vi "Main (NoVisionRequired).vi"() -> ()   [LabVIEW 2019]
uses:
  3D utilities/3DS Models.ctl
  typedefs/System States.ctl
  typedefs/Render States.ctl
  <vilib>/picture/3D Picture Control/Old 3D Toolkit.llb/model.ctl
  <vilib>/picture/3D Picture Control/Old 3D Toolkit.llb/point3f.ctl
  <vilib>/picture/3D Picture Control/Old 3D Toolkit.llb/VertexMode.ctl
  XRay Cabinet/XRay Cabinet.lvclass
  C:/Users/Andrey/Documents/GitHub/XRaySimulatorLV/XRay Scene/XRay Scene.lvclass
  XRay Beam/XRay Beam.lvclass
  XRay CArm/XRay CArm.lvclass
  XRay Part Sample/XRay Part Sample.lvclass
  XRay Table/XRay Table.lvclass
  XRay Beam/XRay Beam.lvclass/XRay Beam.ctl
  XRay Part Sample/XRay Part Sample.lvclass/XRay Part Sample.ctl
  XRay Table/XRay Table.lvclass/XRay Table.ctl
  <vilib>/Analysis/coordinate.llb/3D Cartesian Coordinate Rotation (Euler) (Scalar).vi
  67ea9b9f-5008-4843-b879-74d7c71b0f0c.vi
  XRay Axis Rails/XRay Axis Rails.lvclass
  <vilib>/picture/3D Picture Control/Object/Create Object.vi
  <vilib>/picture/3D Picture Control/Object/Create Object (name).vi
  <vilib>/picture/3D Picture Control/Geometries/Create 3D Axis.vi
  <vilib>/picture/3D Picture Control/Object/Add Object.vi
  <vilib>/picture/3D Picture Control/Object/Add Object (no reference).vi
  XRay Scene/XRay Scene.lvclass
  <vilib>/Analysis/NI_AALPro.lvlib
  3D utilities/3D utilities.lvlib
  <vilib>/picture/3D Picture Control/NI_Old 3D Toolkit.lvlib
  LV_3D_Util64.dll
panel:
  out "XRay Image":sgl[][](graph)
  in  "Link to Z":bool
  in  "Mode":T1(ring)=enum."Wireframe"
  in  "High Res Render":bool
  in  "Play Button":bool
  in  "Reset":bool
  out "Render":bool
  in  "stop":bool
  in  "Part Angle":dbl(knob) caption="Part\nAngle"
  in  "Model":T2
  in  "FDD":sgl(slide)=11.031496 scale=1.0..15.0
  in  "DDA SIZE":sgl(slide)=2.003937 scale=1.0..4.0
  out "Size":i32=1240
  out "Time, ms":dbl=63.153
  out "Max Thickness":sgl=0.5478592
  in  "Y Position":dbl(slide)=7.0 scale=1.0..12.0
  in  "X Position":dbl(slide)=0.5 scale=-2.0..2.0
  in  "C Arm Angle":dbl(knob) caption="C-Arm\nAngle" scale=90.0..-90.0
  in  "Z position":sgl(slide)=4.0 scale=0.0..10.0
  out "3D Picture":refnum<vi>(3d-picture)
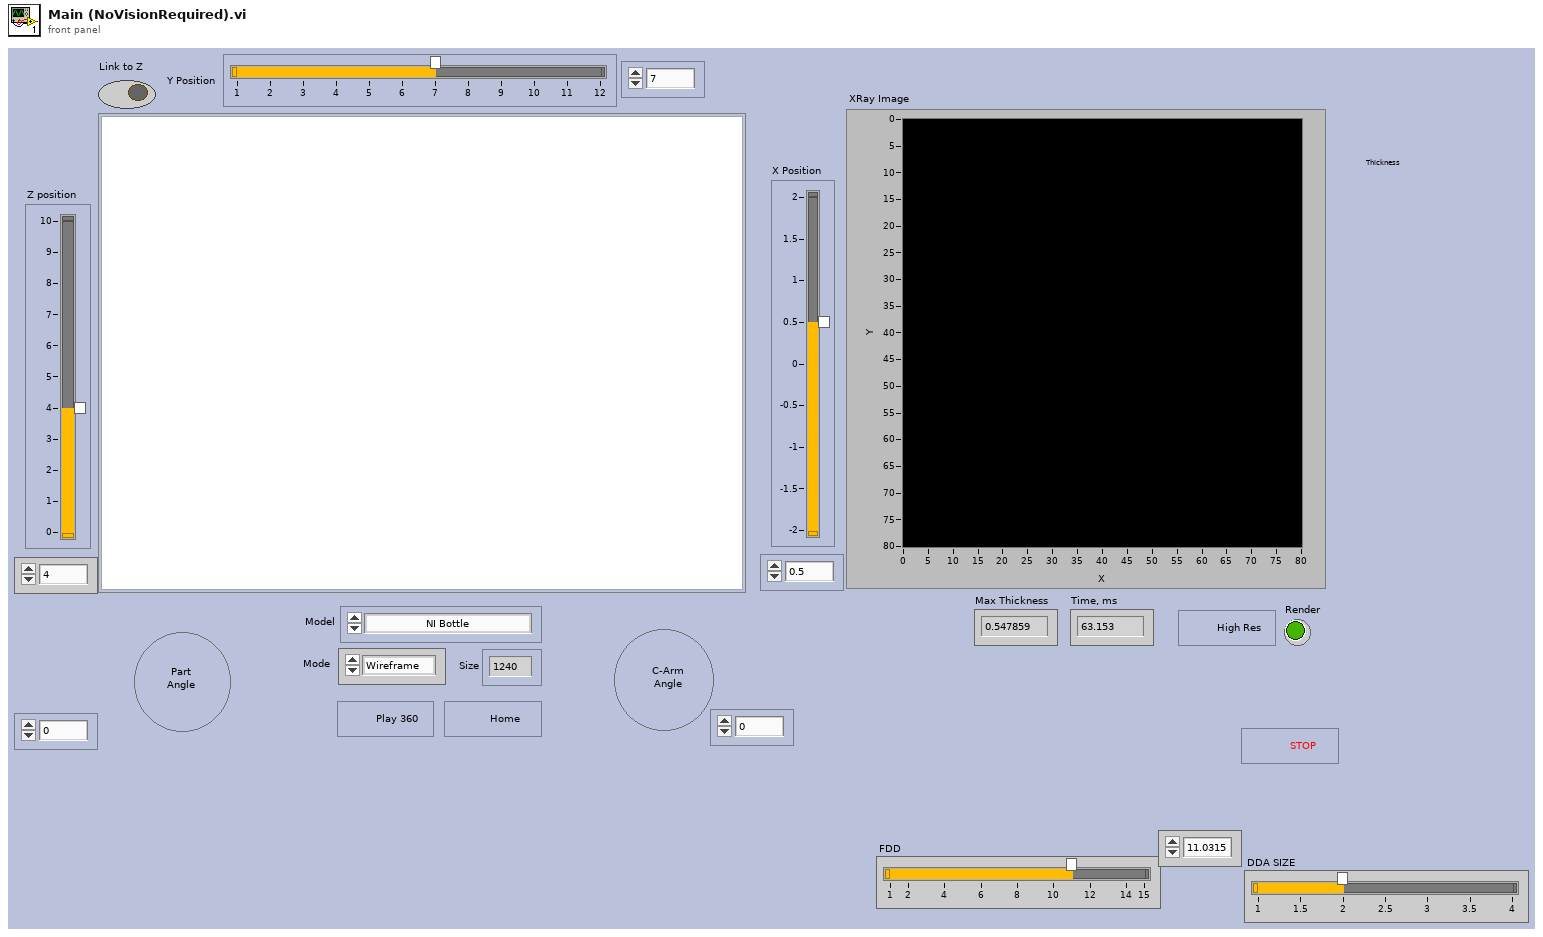
[diagram p1: front panel]
types:
  T1 = enum16{"Inherit Value", "Points", "Wireframe", "Polygons"}
  T2 = typedef "3DS Models.ctl" = enum16{"NI Bottle", "Utah Teapot", "Utah Teapot (Low Res)", "My Cube", "Tree", "Tree 2", "FreeCAD Sample", "Schenkel", "Bunny"}
  T3 = typedef "Render States.ctl" = enum16{"Init", "Create Model", "Move Model", "Render Model", "Render Model (High Res)", "Waiting for Command"}
  T4 = typedef "System States.ctl" = enum16{"Init", "Render", "Waiting for Notification", "Move", "Move 2D Model", "Close and reopen Model", "Quit"}
  T5 = typedef "NI_3D Picture Control.lvlib/NI_Old 3D Toolkit.lvlib/point3f.ctl" = cluster{"x":sgl, "y":sgl, "z":sgl}
  T6 = cluster{"XRay Cabinet":refnum<class "XRay Cabinet.lvclass">, "XRay Beam":refnum<class "XRay Beam.lvclass">, "XRay CArm":refnum<class "XRay CArm.lvclass">, "XRay Part Sample":refnum<class "XRay Part Sample.lvclass">, "XRay Table":refnum<class "XRay Table.lvclass">}
  T7 = typedef "NI_3D Picture Control.lvlib/NI_Old 3D Toolkit.lvlib/model.ctl" = cluster{"VertexList":T5[], "FaceList":cluster{"v1":i32, "v2":i32, "v3":i32}[], "NormalList":T5[], "Mode":T8}
  T8 = typedef "NI_3D Picture Control.lvlib/NI_Old 3D Toolkit.lvlib/VertexMode.ctl" = enum16{"GL_POINTS", "GL_LINES", "GL_LINE_LOOP", "GL_LINE_STRIP", "GL_TRIANGLES", "GL_TRIANGLE_STRIP", "GL_TRIANGLE_FAN", "GL_QUADS", "GL_QUAD_STRIP", "GL_POLYGON"}
  T9 = cluster{"Model":T7, "Vertex":T5[], "FaceList":cluster{"v1":i32, "v2":i32, "v3":i32}[]}
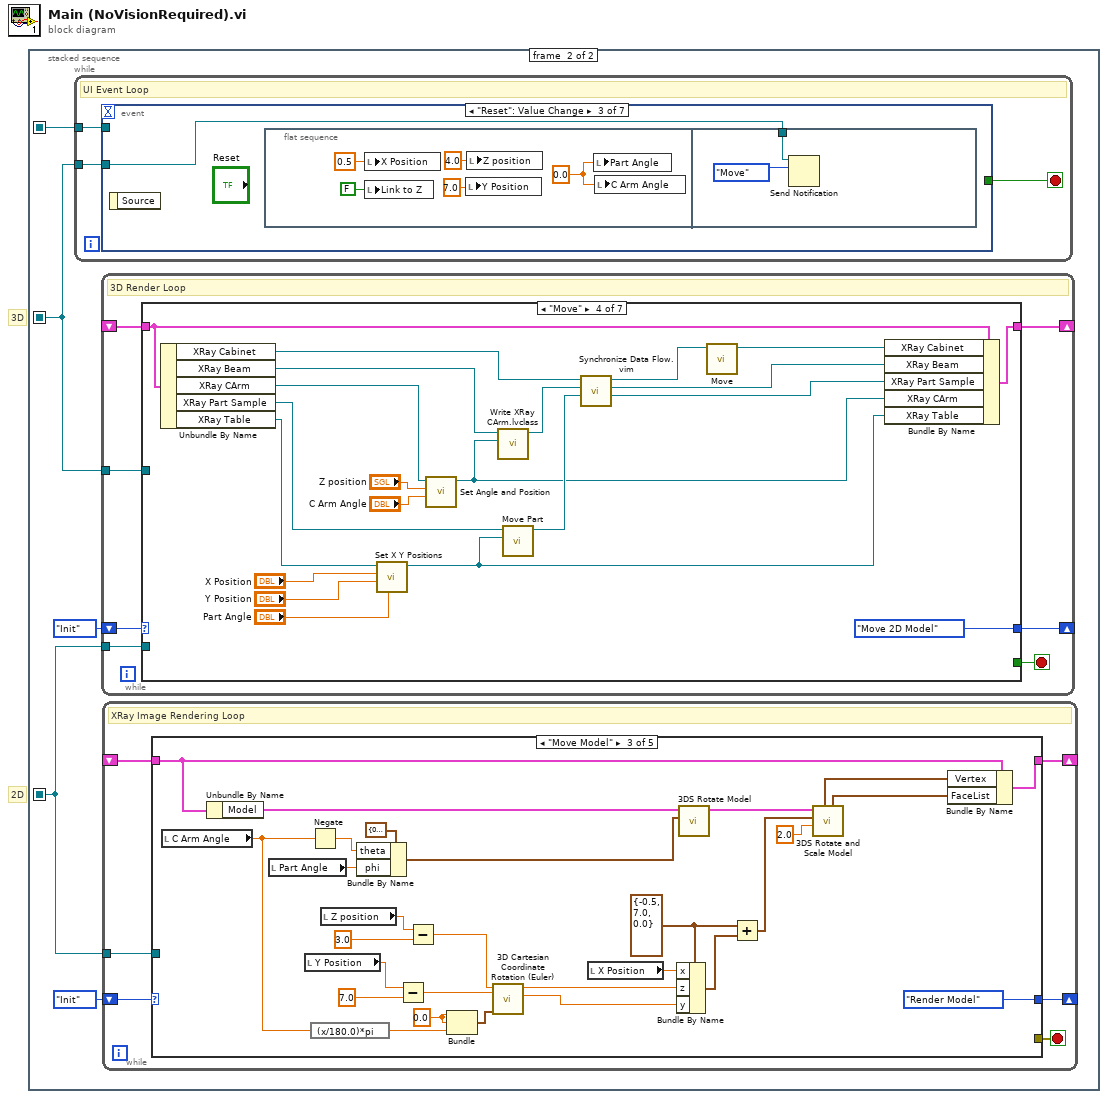
[diagram p0: block diagram]
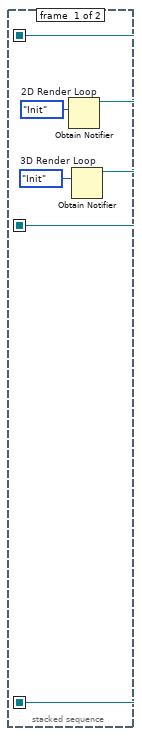
[diagram p2: hidden frame]
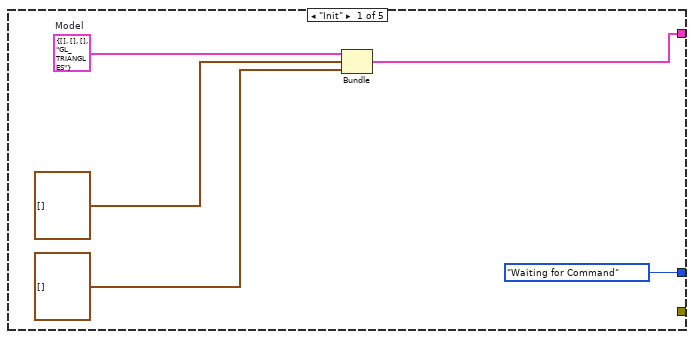
[diagram p3: hidden frame]
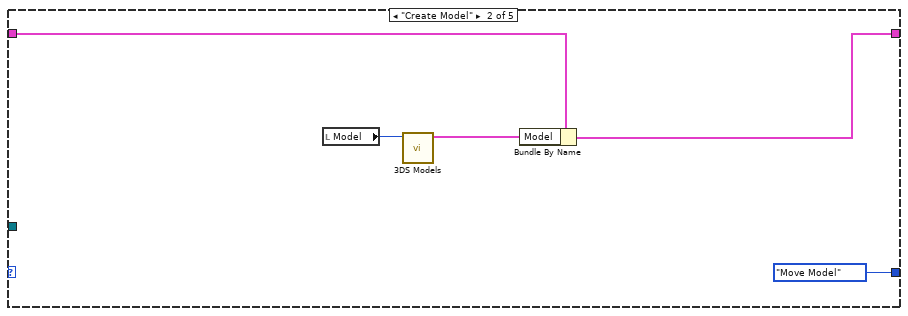
[diagram p4: hidden frame]
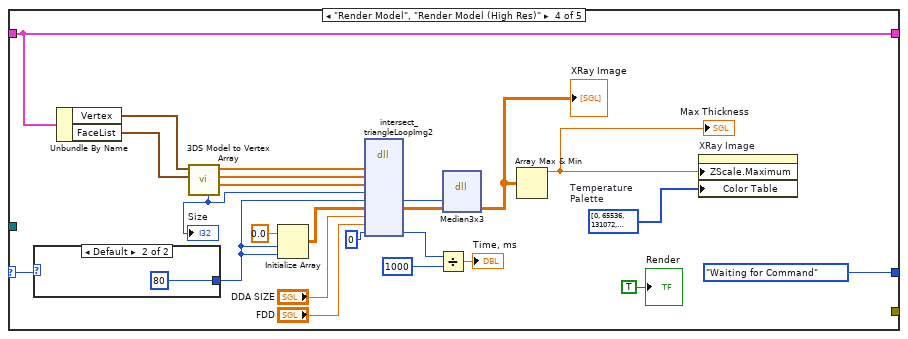
[diagram p5: hidden frame]
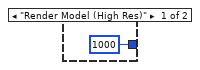
[diagram p6: hidden frame]
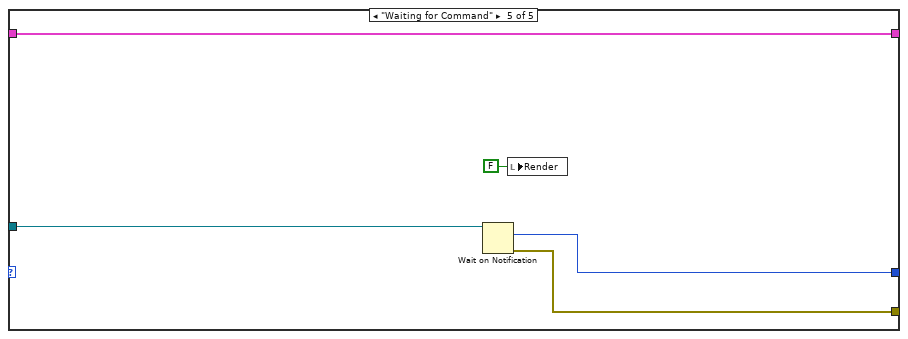
[diagram p7: hidden frame]
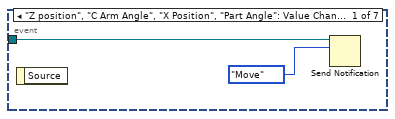
[diagram p8: hidden frame]
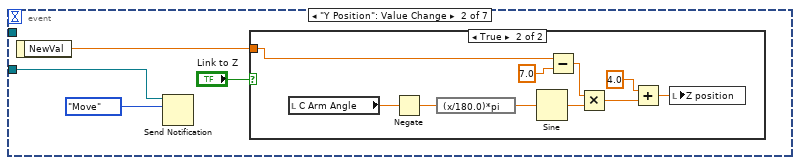
[diagram p9: hidden frame]
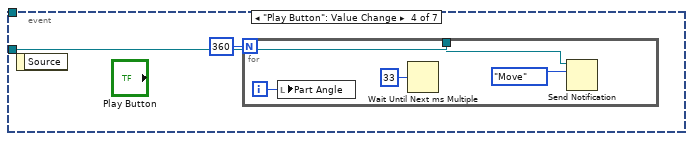
[diagram p11: hidden frame]
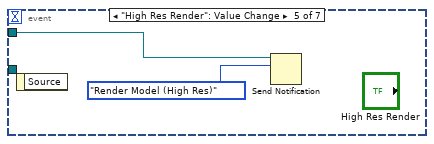
[diagram p12: hidden frame]
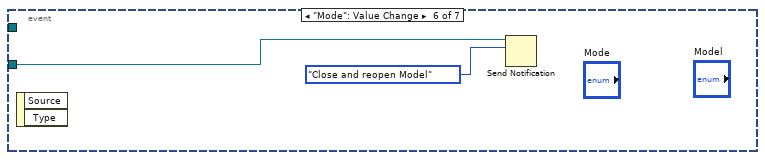
[diagram p13: hidden frame]
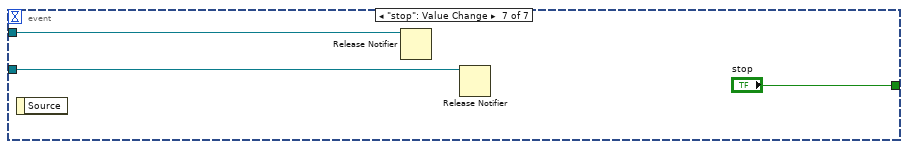
[diagram p14: hidden frame]
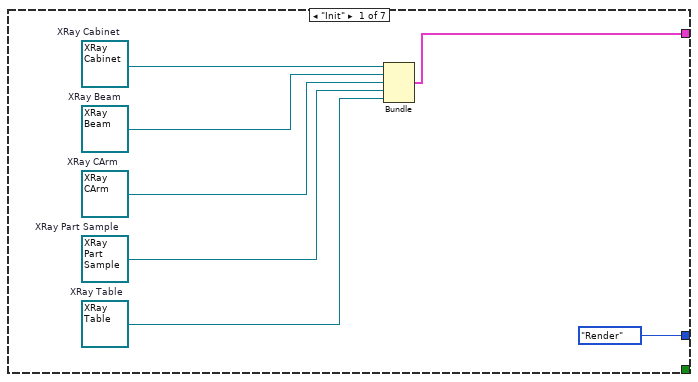
[diagram p15: hidden frame]
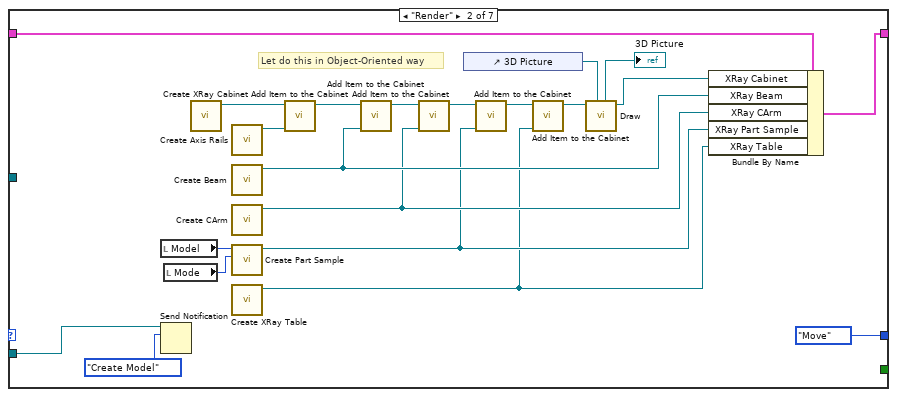
[diagram p16: hidden frame]
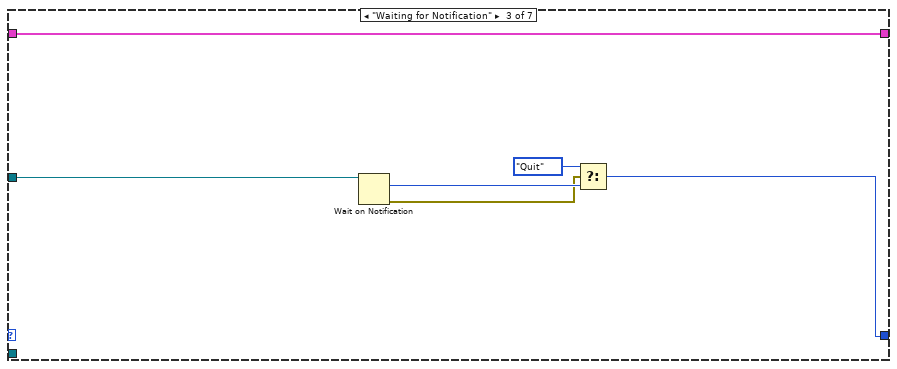
[diagram p17: hidden frame]
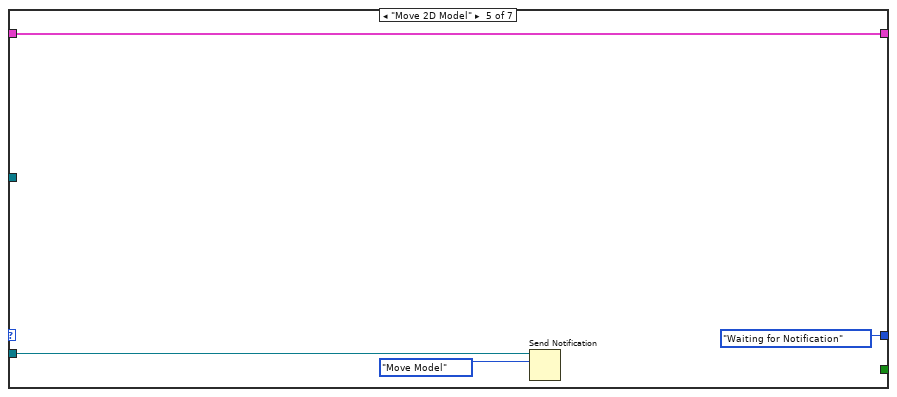
[diagram p18: hidden frame]
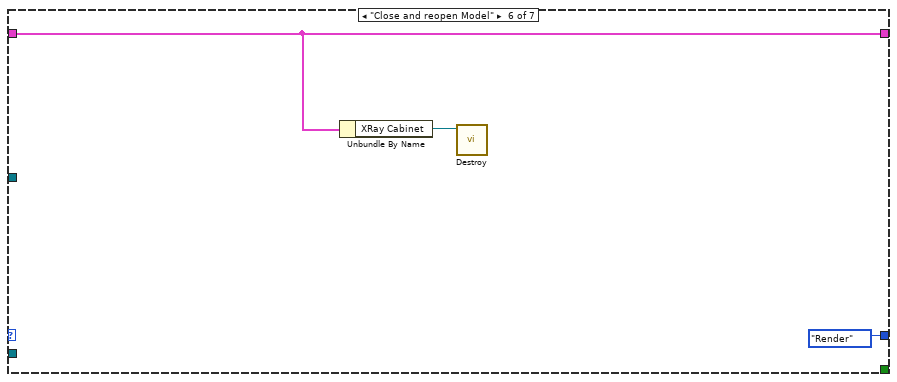
[diagram p19: hidden frame]
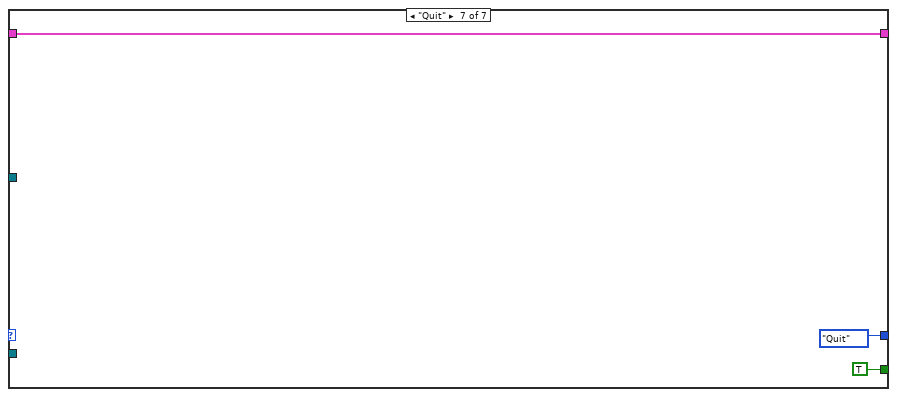
[diagram p20: hidden frame]
diagram:
  # "3D"
  # "2D"
  n1 = stacked-sequence {
    seq-local: [w2 _] -> [_ w5]
    seq-local: [w1 _] -> [_ w7]
    seq-local: [w1 _] -> [_ w6]
    frame #0 {
      w4 = Render_States."Init"  # 2D Render Loop
      w3 = System_States."Init"  # 3D Render Loop
      n2 = Obtain Notifier(notification data type=w4) -> (notifier out=w1:refnum<notifier>)  [unwired: 2 in, 3 out]
      n3 = Obtain Notifier(notification data type=w3) -> (notifier out=w2:refnum<notifier>)  [unwired: 2 in, 3 out]
    }
    frame #1 {
      n4 = while {
        tunnel: w6 -> [w86]
        tunnel: w5 -> [w85]
        stop <- w87 stop-if-true
        # "UI Event Loop"
        n5 = event shown="[2] \"Reset\": Value Change" {
          selector: _ -> [_ _ _ _ _ _ _]
          dyn-events: _ -> [_ _ _ _ _ _ _]
          timeout: _ -> [_ _ _ _ _ _ _]
          tunnel: w85 -> [w89 w92 w104 w112 _ w120 w123]
          tunnel: [_ _ _ _ _ _ "stop"] -> w87
          tunnel: w86 -> [_ _ _ _ w119 _ w122]
          event "Z position", "C Arm Angle", "X Position", "Part Angle": Value Change {
            n6 = event-data() -> ()  [unwired: 1 in, 1 out]
            n7 = Send Notification(notification=System_States."Move", notifier=w89) -> ()  [unwired: 1 in, 2 out]
          }
          event "Y Position": Value Change {
            n8 = event-data() -> ("NewVal"=w91:dbl)  [unwired: 1 in]
            n9 = Send Notification(notification=System_States."Move", notifier=w92) -> ()  [unwired: 1 in, 2 out]
            n10 = case shown="True" "Link to Z" {
              tunnel: w91 -> [_ w98]
              frame False {
              }
              frame True {
                n11 = local read "C Arm Angle"() -> (w101:dbl)
                n12 = Negate(x=w101) -> (-x=w100:dbl)
                n13 = expression code="(x/180.0)*pi" ("degrees to radians")(w100) -> (w99:dbl)
                n14 = Sine(x=w99) -> (sin(x)=w94:dbl)
                n15 = Subtract(x=w98, y=7.0) -> (x-y=w96:dbl)
                n16 = Multiply(x=w96, y=w94) -> (x*y=w95:dbl)
                n17 = Add(x=4.0, y=w95) -> (x+y=w102:dbl)
                n18 = local write "Z position"(w102) -> ()
              }
            }
          }
          event "Reset": Value Change {
            n19 = event-data() -> ()  [unwired: 1 in, 1 out]
            n20 = flat-sequence {
              tunnel: w104 -> [w111]
              frame #0 {
                w106 = 0.0 ("Part Angle")
                n21 = local write "X Position"(0.5 ("X Position")) -> ()
                n22 = local write "Link to Z"(FALSE ("Link to Z")) -> ()
                n23 = local write "Y Position"(7.0 ("Y Position")) -> ()
                n24 = local write "Z position"(sgl 4.0 ("Z position")) -> ()
                n25 = local write "Part Angle"(w106) -> ()
                n26 = local write "C Arm Angle"(w106) -> ()
              }
              frame #1 {
                n27 = Send Notification(notification=System_States."Move", notifier=w111) -> ()  [unwired: 1 in, 2 out]
              }
            }
          }
          event "Play Button": Value Change {
            n28 = event-data() -> ()  [unwired: 1 in, 1 out]
            n29 = for {
              N: 360 -> [_]
              tunnel: w112 -> [w115]
              i -> [w117]
              n30 = local write "Part Angle"(w117) -> ()
              n31 = Wait Until Next ms Multiple(millisecond multiple=u32 33) -> ()  [unwired: 1 out]
              n32 = Send Notification(notification=System_States."Move", notifier=w115) -> ()  [unwired: 1 in, 2 out]
            }
          }
          event "High Res Render": Value Change {
            n33 = event-data() -> ()  [unwired: 1 in, 1 out]
            n34 = Send Notification(notification=Render_States."Render Model (High Res)", notifier=w119) -> ()  [unwired: 1 in, 2 out]
          }
          event "Mode": Value Change {
            n35 = event-data() -> ()  [unwired: 1 in, 2 out]
            n36 = Send Notification(notification=System_States."Close and reopen Model", notifier=w120) -> ()  [unwired: 1 in, 2 out]
          }
          event "stop": Value Change {
            n37 = event-data() -> ()  [unwired: 1 in, 1 out]
            n38 = Release Notifier(notifier=w122) -> ()  [unwired: 1 in, 4 out]
            n39 = Release Notifier(notifier=w123) -> ()  [unwired: 1 in, 4 out]
          }
        }
      }
      n40 = while {
        shift-right: [w130] -> _
        shift-left: System_States."Init" -> [w131]
        shift-right: [w129] -> _
        shift-left: _ -> [w128]
        tunnel: w5 -> [w127]
        tunnel: w7 -> [w125]
        stop <- w126 stop-if-true
        # "3D Render Loop"
        n41 = case shown="\"Move\"" w131 {
          tunnel: [System_States."Render" System_States."Move" w161 System_States."Move 2D Model" System_States."Waiting for Notification" System_States."Render" System_States."Quit"] -> w130
          tunnel: [w132 w144 w165 w170 w187 w192 w194] -> w129
          tunnel: w128 -> [_ w150 w165 w174 w187 w192 w194]
          tunnel: w127 -> [_ _ w164 _ _ _ _]
          tunnel: [_ _ _ _ _ _ TRUE] -> w126
          tunnel: w125 -> [_ w141 _ _ w189 _ _]
          frame "Init" {
            w133 = refnum<class "XRay Table.lvclass"> refnum  # XRay Table
            w134 = refnum<class "XRay Part Sample.lvclass"> refnum  # XRay Part Sample
            w135 = refnum<class "XRay CArm.lvclass"> refnum  # XRay CArm
            w136 = refnum<class "XRay Beam.lvclass"> refnum  # XRay Beam
            w137 = refnum<class "XRay Cabinet.lvclass"> refnum  # XRay Cabinet
            n42 = Bundle("XRay Cabinet"=w137, "XRay Beam"=w136, "XRay CArm"=w135, "XRay Part Sample"=w134, "XRay Table"=w133) -> (w132:T6)  [unwired: 1 in]
          }
          frame "Render" {
            # "Let do this in Object-Oriented way"
            n43 = local read "Model"() -> (w142:T2)
            n44 = Send Notification(notification=Render_States."Create Model", notifier=w141) -> ()  [unwired: 1 in, 2 out]
            n45 = local read "Mode"() -> (w139:T1)
            n46 = call "Create XRay Cabinet.vi"() -> ("XRay Cabinet out"=w154:refnum<class "XRay Cabinet.lvclass">)  [unwired: 10 in, 1 out]
            n47 = call "Create Axis Rails.vi"() -> ("XRay Axis Rails out"=w152:refnum<class "XRay Axis Rails.lvclass">)  [unwired: 10 in, 1 out]
            n48 = call "Create Beam.vi"() -> ("XRay Beam out"=w148:refnum<class "XRay Beam.lvclass">)  [unwired: 10 in, 1 out]
            n49 = call "Create CArm.vi"() -> ("XRay CArm out"=w147:refnum<class "XRay CArm.lvclass">)  [unwired: 10 in, 1 out]
            n50 = call "Create Part Sample.vi"("Draw Style:Mode"=w139, "Model"=w142) -> ("XRay Part Sample out"=w146:refnum<class "XRay Part Sample.lvclass">)  [unwired: 8 in, 1 out]
            n51 = call "Create XRay Table.vi"() -> ("XRay Table out"=w145:refnum<class "XRay Table.lvclass">)  [unwired: 10 in, 1 out]
            n52 = call "Add Item to the Cabinet.vi"("Object"=w152, "XRay Cabinet In"=w154) -> ("XRay Cabinet Out"=w151:refnum<class "XRay Cabinet.lvclass">)  [unwired: 9 in]
            n53 = call "Add Item to the Cabinet.vi"("Object"=w148, "XRay Cabinet In"=w151) -> ("XRay Cabinet Out"=w155:refnum<class "XRay Cabinet.lvclass">)  [unwired: 9 in]
            n54 = call "Add Item to the Cabinet.vi"("Object"=w147, "XRay Cabinet In"=w155) -> ("XRay Cabinet Out"=w157:refnum<class "XRay Cabinet.lvclass">)  [unwired: 9 in]
            n55 = control-ref of="3D Picture"() -> (w153:refnum<vi>)
            n56 = call "Add Item to the Cabinet.vi"("Object"=w146, "XRay Cabinet In"=w157) -> ("XRay Cabinet Out"=w158:refnum<class "XRay Cabinet.lvclass">)  [unwired: 9 in]
            n57 = call "Add Item to the Cabinet.vi"("Object"=w145, "XRay Cabinet In"=w158) -> ("XRay Cabinet Out"=w156:refnum<class "XRay Cabinet.lvclass">)  [unwired: 9 in]
            n58 = call "Draw.vi"("3D Picture"=w153, "XRay Scene in"=w156) -> ("XRay Scene out"=w149:refnum<class "XRay Cabinet.lvclass">, "Scene Object"=→"3D Picture":refnum<vi>)  [unwired: 7 in, 1 out]
            n59 = Bundle By Name(cluster=w150, "XRay Cabinet"=w149, "XRay Beam"=w148, "XRay CArm"=w147, "XRay Part Sample"=w146, "XRay Table"=w145) -> (w144:T6)
          }
          frame "Waiting for Notification" {
            n60 = Wait on Notification(notifier=w164) -> (notification=w163:T4, error out=w162:errorcluster)  [unwired: 1 in, 4 out]
            n61 = Select(t=System_States."Quit", s=w162, f=w163) -> (s? t:f=w161:T4)
          }
          frame "Move" {
            n62 = Unbundle By Name(w174) -> ("XRay Cabinet"=w179:refnum<class "XRay Cabinet.lvclass">, "XRay Beam"=w178:refnum<class "XRay Beam.lvclass">, "XRay CArm"=w177:refnum<class "XRay CArm.lvclass">, "XRay Part Sample"=w176:refnum<class "XRay Part Sample.lvclass">, "XRay Table"=w175:refnum<class "XRay Table.lvclass">)
            n63 = call "Set X Y Positions.vi"("Table Rotation"="Part Angle", "Y Position"="Y Position", "X Position"="X Position", "XRay Table in"=w175) -> ("XRay Table out"=w167:refnum<class "XRay Table.lvclass">)  [unwired: 6 in, 1 out]
            n64 = call-dynamic "Set Angle and Position.vi"("Angle"="C Arm Angle", "Z"="Z position", "XRay CArm in"=w177) -> ("XRay CArm out"=w168:refnum<class "XRay CArm.lvclass">)  [unwired: 7 in, 1 out]
            n65 = call "Write XRay CArm.lvclass.vi"("XRay CArm.lvclass"=w168, "XRay Beam in"=w178) -> ("XRay Beam out"=w181:refnum<class "XRay Beam.lvclass">)  [unwired: 8 in, 1 out]
            n66 = call "Move Part.vi"("XRay Table.lvclass"=w167, "XRay Part Sample in"=w176) -> ("XRay Part Sample out"=w171:refnum<class "XRay Part Sample.lvclass">)  [unwired: 8 in, 1 out]
            n67 = call "Synchronize Data Flow.vim"("input 3"=w171, "input 2"=w181, "input 1"=w179) -> ("output 3"=w169:refnum<class "XRay Part Sample.lvclass">, "output 2"=w172:refnum<class "XRay Beam.lvclass">, "output 1"=w182:refnum<class "XRay Cabinet.lvclass">)  [unwired: 1 in, 1 out]
            n68 = call-dynamic "Move.vi"("XRay Scene in"=w182) -> ("XRay Scene out"=w173:refnum<class "XRay Cabinet.lvclass">)  [unwired: 8 in, 2 out]
            n69 = Bundle By Name(cluster=w174, "XRay Cabinet"=w173, "XRay Beam"=w172, "XRay Part Sample"=w169, "XRay CArm"=w168, "XRay Table"=w167) -> (w170:T6)
          }
          frame "Move 2D Model" {
            n70 = Send Notification(notification=Render_States."Move Model", notifier=w189) -> ()  [unwired: 1 in, 2 out]
          }
          frame "Close and reopen Model" {
            n71 = Unbundle By Name(w192) -> ("XRay Cabinet"=w191:refnum<class "XRay Cabinet.lvclass">)
            n72 = call-dynamic "Destroy.vi"("XRay Cabinet in"=w191) -> ()  [unwired: 9 in, 2 out]
          }
          frame "Quit" {
          }
        }
      }
      n73 = while {
        shift-right: [w12] -> _
        shift-left: Render_States."Init" -> [w15]
        shift-right: [w14] -> _
        shift-left: _ -> [w13]
        tunnel: w7 -> [w11]
        stop <- w10 stop-if-true
        # "XRay Image Rendering Loop"
        n74 = case shown="\"Move Model\"" w15 {
          selector: w15 -> [_ _ _ w60 _]
          tunnel: [w16 w24 w34 w63 w84] -> w14
          tunnel: w13 -> [_ w25 w35 w63 w84]
          tunnel: [Render_States."Waiting for Command" Render_States."Move Model" Render_States."Render Model" Render_States."Waiting for Command" w82] -> w12
          tunnel: w11 -> [_ _ _ _ w83]
          tunnel: [_ _ _ _ w81] -> w10
          frame "Init" {
            w20 = T7 {"VertexList"=[], "FaceList"=[], "NormalList"=[], "Mode"=enum."GL_TRIANGLES"}  # Model
            n75 = Bundle("Model"=w20, "Vertex"=T5[] [], "FaceList"=cluster{"v1":i32, "v2":i32, "v3":i32}[] []) -> (w16:T9)  [unwired: 1 in]
          }
          frame "Create Model" {
            n76 = local read "Model"() -> (w21:T2)
            n77 = call "3DS Models.vi"("Model"=w21) -> ("Model Out"=w22:T7)  [unwired: 10 in]
            n78 = Bundle By Name(cluster=w25, "Model"=w22) -> (w24:T9)
          }
          frame "Move Model" {
            w31 = T5 {"x"=-0.5, "y"=7.0, "z"=0.0} ("point3f - SHIFT")
            w42 = 0.0 ("x/y")
            n79 = local read "C Arm Angle"() -> (w26:dbl)
            n80 = Unbundle By Name(w35) -> ("Model"=w38:T7)
            n81 = local read "Part Angle"() -> (w53:dbl)
            n82 = local read "Y Position"() -> (w48:dbl)
            n83 = Negate(x=w26) -> (-x=w49:dbl)
            n84 = expression code="(x/180.0)*pi" ("degrees to radians")(w26) -> (w32:dbl)
            n85 = local read "Z position"() -> (w47:sgl)
            n86 = Bundle By Name(cluster=cluster{"phi":dbl, "theta":dbl, "psi":dbl} {"phi"=0.0, "theta"=0.0, "psi"=1.0} ("Euler Angles"), "theta"=w49, "phi"=w53) -> (w45:cluster{"phi":dbl, "theta":dbl, "psi":dbl})
            n87 = Subtract(x=w48, y=7.0) -> (x-y=w50:dbl)
            n88 = Subtract(x=w47, y=3.0) -> (x-y=w51:dbl)
            n89 = Bundle("x/y"=w42, "x/y"=w42, "C Arm Angle"=w32) -> (w52:cluster{"x/y":dbl, "x/y":dbl, "C Arm Angle":dbl})  [unwired: 1 in]
            n90 = call-poly <vilib>:"3D Cartesian Coordinate Rotation (Euler).vi"("Euler Angles"=w52, "y"=w50, "x"=w51) -> ("y out"=w28:dbl, "x out"=w29:dbl)  [unwired: 5 in, 2 out]
            n91 = local read "X Position"() -> (w30:dbl)
            n92 = Bundle By Name(cluster=w31, "x"=w30, "z"=w29, "y"=w28) -> (w27:T5)
            n93 = call "3DS Rotate Model.vi"("Euler Angles"=w45, "model in"=w38) -> ("model out"=w44:T7)  [unwired: 9 in]
            n94 = Add(x=w31, y=w27) -> (x+y=w46:T5)
            n95 = call "3DS Rotate and Scale Model.vi"("scale"=sgl 2.0, "point3f - SHIFT"=w46, "Object In"=w44) -> ("FaceList"=w36:cluster{"v1":i32, "v2":i32, "v3":i32}[], "Vertex"=w37:T5[])  [unwired: 5 in, 2 out]
            n96 = Bundle By Name(cluster=w35, "Vertex"=w37, "FaceList"=w36) -> (w34:T9)
          }
          frame "Render Model", "Render Model (High Res)" {
            w58 = u32[] [0, 65536, 131072, 196608, 262144, 327680, 393216, 458752, 524288, 589824, 655360, 720896, 786432, 851968, 917504, 983040, 1048576, 1114112, 1179648, 1245184, 1310720, 1376256, 1441792, 1507328, 1572864, 1638400, 1703936, 1769472, 1835008, 1900544, 1966080, 2031616, 2097152, 2162688, 2228224, 2293760, 2359296, 2424832, 2490368, 2555904, 2621440, 2686976, 2752512, 2818048, 2883584, 2949120, 3014656, 3080192, 3145728, 3211264, 3276800, 3342336, 3407872, 3473408, 3538944, 3604480, 3670016, 3735552, 3801088, 3866624, 3932160, 3997696, 4063232, 4128768, 4194304, 4259840, 4325376, 4390912, 4456448, 4521984, 4587520, 4653056, 4718592, 4784128, 4849664, 4915200, 4980736, 5046272, 5111808, 5177344, 5242880, 5308416, 5373952, 5439488, 5505024, 5570560, 5636096, 5701632, 5767168, 5832704, 5898240, 5963776, 6029312, 6094848, 6160384, 6225920, 6291456, 6356992, 6422528, 6488064, 6553600, 6619136, 6684672, 6750208, 6815744, 6881536, 6947584, 7013632, 7079424, 7145472, 7211520, 7277312, 7343360, 7409408, 7475200, 7541248, 7607296, 7673088, 7739136, 7805184, 7871232, 7937024, 8003072, 8069120, 8134912, 8200960, 8267008, 8332800, 8398848, 8464896, 8530688, 8596736, 8662784, 8728576, 8794624, 8860672, 8926720, 8992512, 9058560, 9124608, 9190400, 9256448, 9322496, 9388290, 9454340, 9520390, 9586185, 9652235, 9718285, 9784079, 9850130, 9916180, 9982230, 10048024, 10114075, 10180125, 10245919, 10311969, 10378020, 10443814, 10509864, 10575914, 10641709, 10707759, 10773809, 10839859, 10905654, 10971704, 11037754, 11103548, 11169599, 11235649, 11301443, 11367493, 11433544, 11499338, 11565388, 11631438, 11697233, 11763283, 11829333, 11895384, 11961178, 12027228, 12093278, 12159073, 12225123, 12291173, 12356967, 12423018, 12489068, 12554862, 12620912, 12686963, 12752757, 12818807, 12884857, 12950908, 13016702, 13082752, 13148802, 13214597, 13280647, 13346697, 13412491, 13478542, 13544592, 13610386, 13676436, 13742487, 13808537, 13874331, 13940381, 14006432, 14072226, 14138276, 14204326, 14270121, 14336171, 14402221, 14468016, 14534066, 14600116, 14665910, 14731961, 14798011, 14864061, 14929855, 14995906, 15061956, 15127750, 15193800, 15259851, 15325645, 15391695, 15457745, 15523540, 15589590, 15655640, 15721434, 15787485, 15853535, 15919585, 15985379, 16051430, 16117480, 16183274, 16249324, 16315375, 16381169, 16447219, 16513269, 16579064, 16645114, 16711164, 16777215]  # Temperature Palette
            n97 = case shown="Default" w60 {
              tunnel: [1000 ("IMAGE SIZE") 80 ("IMAGE SIZE")] -> w59
              frame "Render Model (High Res)" {
              }
              frame Default {
              }
            }
            n98 = Unbundle By Name(w63) -> ("Vertex"=w65:T5[], "FaceList"=w64:cluster{"v1":i32, "v2":i32, "v3":i32}[])
            n99 = call "3DS Model to Vertex Array.vi"("FaceList"=w64, "Array"=w65) -> ("point3f 2"=w72:sgl[], "point3f 3"=w71:sgl[], "point3f"=w74:sgl[], "Count"=w75:i32)  [unwired: 6 in]
            "Size" <- w75
            n100 = Initialize Array(sgl 0.0 ("element"), w59, w59) -> (w73:sgl[][])
            n101 = dll-call lib="C:/Users/Andrey/Documents/GitHub/XRaySimulatorLV/LV_3D_Util*.*" fn="intersect_triangleLoopImg2" ("LV_3D_Util.dll:\nintersect_\ntriangleL\noopImg2")("vert0"=w74, "vert1"=w71, "vert2"=w72, "MeshSize"=w75, "ImageSize"=w59, "image"=w73, "DetectorSize"="DDA SIZE", "FDD"="FDD", "Execution Time"=u64 0) -> ("ImageSize"=w56:i32, "image"=w57:sgl[][], "Execution Time"=w76:u64)  [unwired: 10 in, 2 out]
            n102 = Divide(x=w76, y=u64 1000) -> (x/y=→"Time, ms":dbl)
            n103 = dll-call lib="C:/Users/Andrey/Documents/GitHub/XRaySimulatorLV/LV_3D_Util*.*" fn="Median3x3" ("LV_3D_Util.dll:\nintersect_\ntriangleL\noopImg2")("ImageSize"=w56, "image"=w57) -> ("image"=w55:sgl[][])  [unwired: 5 in, 2 out]
            "XRay Image" <- w55
            n104 = Array Max & Min(array=w55) -> (max value=w54:sgl)  [unwired: 3 out]
            "Max Thickness" <- w54
            n105 = property on="XRay Image" class="IntGraph (strict)"("ZScale.Maximum"=w54, "Color Table"=w58) -> ()  [unwired: 2 in, 2 out]
            "Render" <- TRUE ("Render")
          }
          frame "Waiting for Command" {
            n106 = Wait on Notification(notifier=w83) -> (notification=w82:T3, error out=w81:errorcluster)  [unwired: 1 in, 4 out]
            n107 = local write "Render"(FALSE ("Render")) -> ()
          }
        }
      }
    }
  }
